vi "Bunch_points.vi"() -> ()   [LabVIEW 2011]
uses:
  <vilib>/Utility/file.llb/Read From Spreadsheet File (DBL).vi
panel:
  out "Pivot point":cluster{"R":dbl, "S":dbl, "T":dbl}
  in  "stop":bool
  in  "Log time (sec)":dbl=3.0
  out "points done":i32
  out "Status":string
  out "Move possible":bool
  out "Diagnostics ASAP":cluster{"Valid position":bool, "Message":string}
  in  "Ouput reference file":path=path "C:/Documents and Settings/ram/My Documents/work/asap/cal_data/new/calibration_ref.dat"
  out "# Points":i32
  in  "Input points path":path=path "C:/Documents and Settings/ram/My Documents/work/asap/cal_data/hex39/goals_trans.dat"
  out "Moving?":bool
  in  "Velocity values":dbl[](array[numeric])=[2.0] format="%.4f"
  out "Position":dbl[](array[numeric]) format="%.4f"
  out "Conn. Axes":string[](array[string])
  out "Identification":string
  out "Hexapod initialized?":bool
  # "HEXAPOD CONTROL"
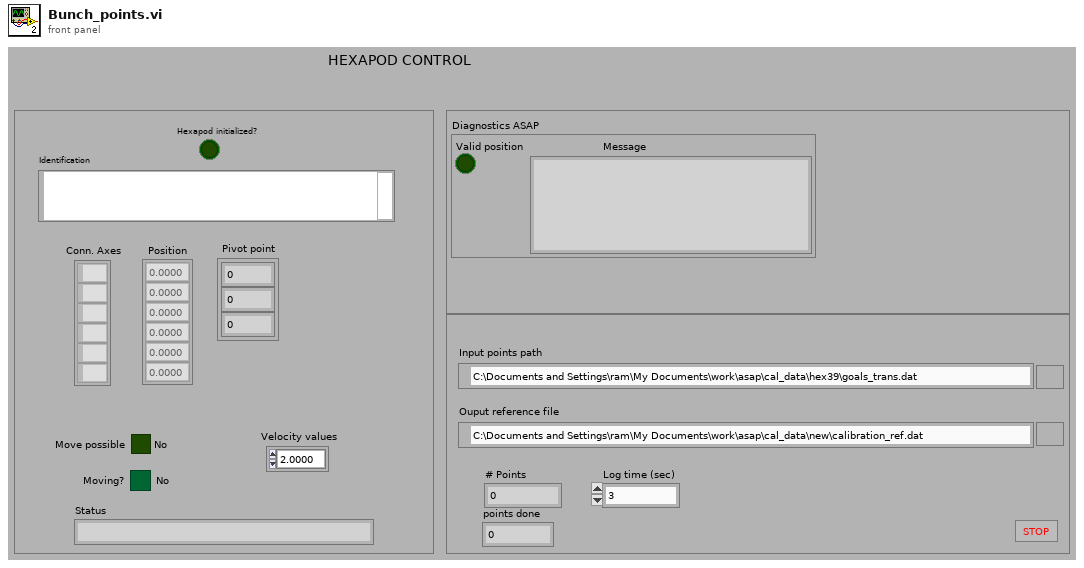
[diagram p1: front panel]
types:
  T1 = enum16{"open", "replace", "create", "open or create", "replace or create", "replace or create with confirmation"}
  T2 = cluster{"all rows[0]":dbl, "all rows[1]":dbl, "all rows[2]":dbl}
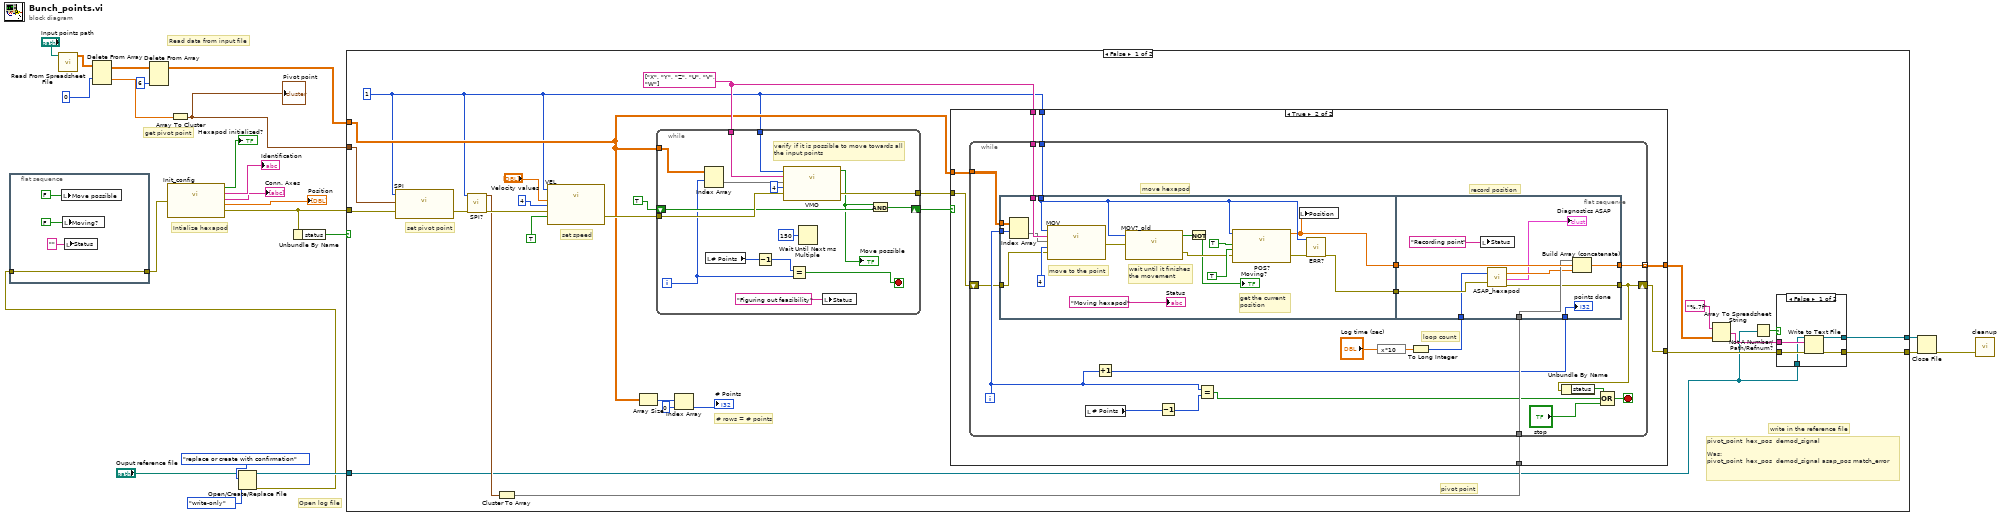
[diagram p0: block diagram]
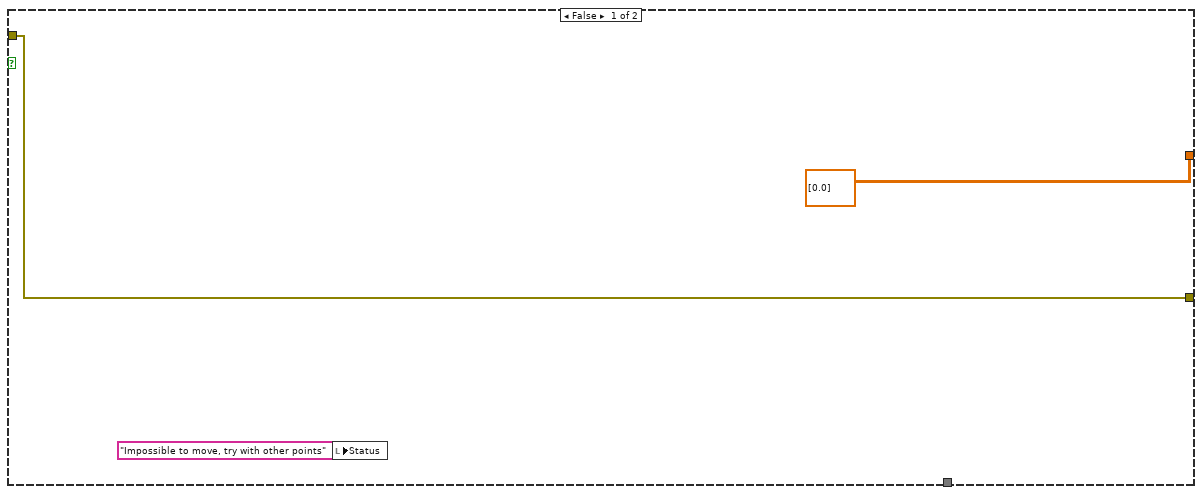
[diagram p3: hidden frame]
diagram:
  # "Read data from input file"
  # "Intialize hexapod"
  # "get pivot point"
  # "Open log file"
  n1 = flat-sequence {
    tunnel: w4 -> [w24]
    tunnel: [w24] -> w3
    frame #0 {
      n2 = local write "Move possible"(FALSE ("Move possible")) -> ()
      n3 = local write "Moving?"(FALSE ("Moving?")) -> ()
      n4 = local write "Status"("" ("Status")) -> ()
    }
  }
  n5 = call-poly <vilib>:"Read From Spreadsheet File.vi"("file path (dialog if empty)"="Input points path") -> ("all rows"=w11:dbl[][])  [unwired: 6 in, 4 out]
  n6 = Delete From Array(array=w11, index (row)=0) -> (deleted portion=w1:dbl[], array with subset deleted=w10:dbl[][])  [unwired: 2 in]
  n7 = Delete From Array(array=w10, index (col)=6 ("disabled index (col)")) -> (array with subset deleted=w9:dbl[][])  [unwired: 2 in, 1 out]
  n8 = call "Init_config.vi"("error in"=w3) -> ("Hexapod initialized?"=→"Hexapod initialized?":bool, "Identification"=→"Identification":string, "Conn. Axes"=→"Conn. Axes":string[], "Position"=→"Position":dbl[], "error out"=w19:errorcluster)  [unwired: 10 in]
  n9 = Array To Cluster(array=w1) -> (cluster=w2:T2)
  "Pivot point" <- w2
  n10 = Open/Create/Replace File(file path (use dialog)="Ouput reference file", operation (0:open)=T1."replace or create with confirmation", access (0:read/write)=enum16{"read/write", "read-only", "write-only"}."write-only") -> (refnum out=w14:refnum<file>, error out=w4:errorcluster)  [unwired: 3 in, 1 out]
  n11 = Unbundle By Name(w19) -> ("status"=w18:bool)
  n12 = case shown="False" w18 {
    tunnel: w19 -> [w54 w135]
    tunnel: w14 -> [w29 w136]
    tunnel: w9 -> [w39 _]
    tunnel: w2 -> [w37 _]
    tunnel: [w33 w136] -> w7
    tunnel: [w28 w135] -> w5
    frame False {
      w46 = string[] ["X", "Y", "Z", "U", "V", "W"]
      w38 = 1 ("System no.")
      # "write in the reference file"
      # "set speed"
      # "set pivot point"
      # "pivot point"
      # "pivot_point  hex_pos  demod_signal\n\nWas:\npivot_point  hex_pos  demod_signal asap_pos match_error"
      # "# rows = # points"
      n13 = call "SPI.vi"("System no."=w38, "Pivot point coordinates"=w37, "error in"=w54) -> ("error out"=w42:errorcluster)  [unwired: 15 in, 1 out]
      n14 = call "SPI?.vi"("System no."=w38, "error in"=w42) -> ("Pivot point coordinates"=w36:cluster{"R":dbl, "S":dbl, "T":dbl}, "error out"=w41:errorcluster)  [unwired: 16 in]
      n15 = Cluster To Array(cluster=w36) -> (array=w40:dbl[])
      n16 = call "VEL.vi"("System no."=w38, "Velocity values"="Velocity values", "No.of digits"=i16 4, "error in"=w41, "Without axis ID?"=TRUE) -> ("error out"=w50:errorcluster)  [unwired: 13 in, 1 out]
      n17 = Array Size(array=w39) -> (size(s)=w45:i32[])
      n18 = while {
        tunnel: w38 -> [w77]
        tunnel: w46 -> [w75]
        tunnel: w50 -> [w73]
        tunnel: [w72] -> w47
        shift-right: [w71] -> w48
        shift-left: TRUE ("x") -> [w70]
        tunnel: w39 -> [w69]
        i -> [w67]
        stop <- w66 stop-if-true
        # "verify if it is possible to move towards all\nthe input points"
        n19 = Index Array(array=w69, index (row)=w67) -> (element=w76:dbl[])  [unwired: 1 in]
        n20 = local read "# Points"() -> (w65:i32)
        n21 = Decrement(x=w65) -> (x-1=w68:i32)
        n22 = call "VMO.vi"("System no."=w77, "Axes to command"=w75, "Position values"=w76, "No.of digits"=i16 4, "error in"=w73) -> ("Move possible"=w63:bool, "error out"=w72:errorcluster)  [unwired: 13 in]
        "Move possible" <- w63
        n23 = Equal?(x=w68, y=w67) -> (x = y?=w66:bool)
        n24 = Wait Until Next ms Multiple(millisecond multiple=u32 150) -> ()  [unwired: 1 out]
        n25 = local write "Status"("Figuring out feasibility" ("Status")) -> ()
        n26 = And(x=w63, y=w70) -> (x .and. y?=w71:bool)
      }
      n27 = Index Array(array=w45, index=0) -> (element=→"# Points":i32)
      n28 = case shown="True" w48 {
        tunnel: w47 -> [w78 w82]
        tunnel: w38 -> [_ w87]
        tunnel: w46 -> [_ w86]
        tunnel: w39 -> [_ w85]
        tunnel: [dbl[][] [[0.0]] ("1 row output") w83] -> w30
        tunnel: w40 -> [_ w84]
        tunnel: [w78 w81] -> w32
        frame False {
          n29 = local write "Status"("Impossible to move, try with other points" ("Status")) -> ()
        }
        frame True {
          n30 = while {
            tunnel: w87 -> [w103]
            tunnel: w86 -> [w107]
            tunnel: w85 -> [w106]
            tunnel: w84 -> [w102]
            tunnel: [w101] -> w83 mode=indexing
            shift-right: [w96] -> w81
            shift-left: w82 -> [w98]
            i -> [w100]
            stop <- w93 stop-if-true
            # "loop count"
            # "record position"
            # "move hexapod"
            n31 = flat-sequence {
              tunnel: w107 -> [w124]
              tunnel: w103 -> [w118]
              tunnel: w106 -> [w116]
              tunnel: w100 -> [w114]
              tunnel: w98 -> [w112]
              tunnel: [w109] -> w97
              tunnel: [w108] -> w91
              tunnel: w88 -> [w126]
              tunnel: w102 -> [w134]
              tunnel: [w133] -> w101
              tunnel: w99 -> [w130]
              tunnel: w97 -> [w127]
              tunnel: [w129] -> w96
              tunnel: w91 -> [w128]
              frame #0 {
                # "wait until it finishes\nthe movement"
                # "get the current \nposition"
                # "move to the point"
                n32 = Index Array(array=w116, index (row)=w114) -> (element=w111:dbl[])  [unwired: 1 in]
                n33 = call "MOV.vi"("System no."=w118, "Axes to move"=w124, "Position values"=w111, "No.of digits"=i16 4, "error in"=w112) -> ("error out"=w122:errorcluster)  [unwired: 14 in]
                n34 = call "MOV?_old.vi"("System no."=w118, "error in"=w122) -> ("Moving?"=w117:bool, "error out"=w115:errorcluster)  [unwired: 16 in]
                n35 = Not(x=w117) -> (.not. x?=→"Moving?":bool)
                n36 = call "POS?.vi"("System no."=w118, "All axes?"=TRUE, "Axis identifier?"=TRUE, "error in"=w115) -> ("Position"=w108:dbl[], "error out"=w119:errorcluster)  [unwired: 14 in]
                n37 = local write "Position"(w108) -> ()
                n38 = call "ERR?.vi"("System no."=w118, "error in"=w119) -> ("error out"=w109:errorcluster)  [unwired: 16 in, 1 out]
                "Status" <- "Moving hexapod"
              }
              frame #1 {
                n39 = local write "Status"("Recording point" ("Status")) -> ()
                n40 = call "ASAP_hexapod.vi"("Iterations"=w126, "error in"=w127) -> ("Demodulated averaged"=w132:sgl[], "Diagnostics ASAP"=→"Diagnostics ASAP":cluster{"Valid position":bool, "Message":string}, "error out"=w129:errorcluster)  [unwired: 15 in]
                n41 = Build Array (concatenate)(w134, w128, w132) -> (w133:dbl[])
                "points done" <- w130
              }
            }
            n42 = local read "# Points"() -> (w105:i32)
            n43 = Increment(x=w100) -> (x+1=w99:i32)
            n44 = Decrement(x=w105) -> (x-1=w104:i32)
            n45 = Equal?(x=w100, y=w104) -> (x = y?=w94:bool)
            n46 = expression code="x*10"("Log time (sec)") -> (w89:dbl)
            n47 = To Long Integer(number=w89) -> (32bit integer=w88:i32)
            n48 = Unbundle By Name(w96) -> ("status"=w95:bool)
            n49 = Compound Arithmetic op=OR(w95, w94, "stop") -> (w93:bool)
          }
        }
      }
      n50 = Array To Spreadsheet String(array=w30, 3:"%.7f" ("format (%.3f)")) -> (spreadsheet string=w34:string)  [unwired: 1 in]
      n51 = Not A Number/Path/Refnum?(number/path/refnum=w29) -> (NaN/Path/Refnum?=w31:bool)
      n52 = case shown="False" w31 {
        tunnel: w34 -> [w59 _]
        tunnel: [w58 w61] -> w33
        tunnel: w32 -> [w57 w60]
        tunnel: [w56 w60] -> w28
        tunnel: w29 -> [w55 w61]
        frame False {
          n53 = Write to Text File(file (use dialog)=w55, text=w59, error in=w57) -> (refnum out=w58:refnum<file>, error out=w56:errorcluster)  [unwired: 1 in, 1 out]
        }
        frame True {
        }
      }
    }
    frame True {
    }
  }
  n54 = Close File(refnum=w7, error in=w5) -> (error out=w6:errorcluster)  [unwired: 1 out]
  n55 = call "cleanup.vi"("error in"=w6) -> ()  [unwired: 2 in, 1 out]
